vi "Top-Level.vi"   [LabVIEW 2012]
uses:
  eventlib/TAS_Event.lvclass
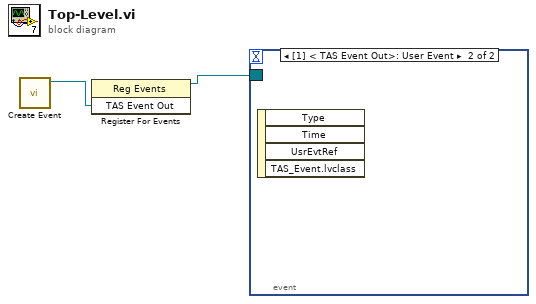
[diagram p0: block diagram]
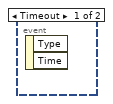
[diagram p2: hidden frame]
diagram:
  n1 = call-dynamic "Create Event.vi"() -> ("TAS Event Out"=w2:refnum<user-event>)  [unwired: 10 in, 1 out]
  n2 = register-events(w2) -> (reference out=w1:refnum<event-registration>)  [unwired: 2 in, 1 out]
  n3 = event shown="[1] <\nTAS Event Out>: User Event" {
    selector: w1 -> [_ _]
    dyn-events: _ -> [_ _]
    timeout: _ -> [_ _]
    event Timeout {
      n4 = event-data() -> ()  [unwired: 1 in, 2 out]
    }
    event User Event {
      n5 = event-data() -> ()  [unwired: 1 in, 4 out]
    }
  }
